vi "YENİİİİİ.vi"() -> ()   [LabVIEW 2018]
uses:
  <vilib>/Instr/_visa.llb/VISA Configure Serial Port (Instr).vi
panel:
  out "humimade":dbl(knob) scale=0.0..100.0
  out "temperature":dbl(slide) scale=0.0..100.0
  out "humimade":i32
  in  "stop":bool
  out "termo":i32
  in  "VISA resource name":refnum<visa-resource-name>
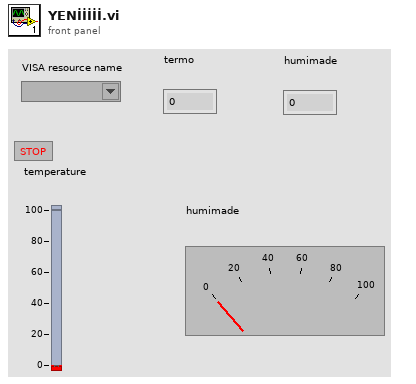
[diagram p1: front panel]
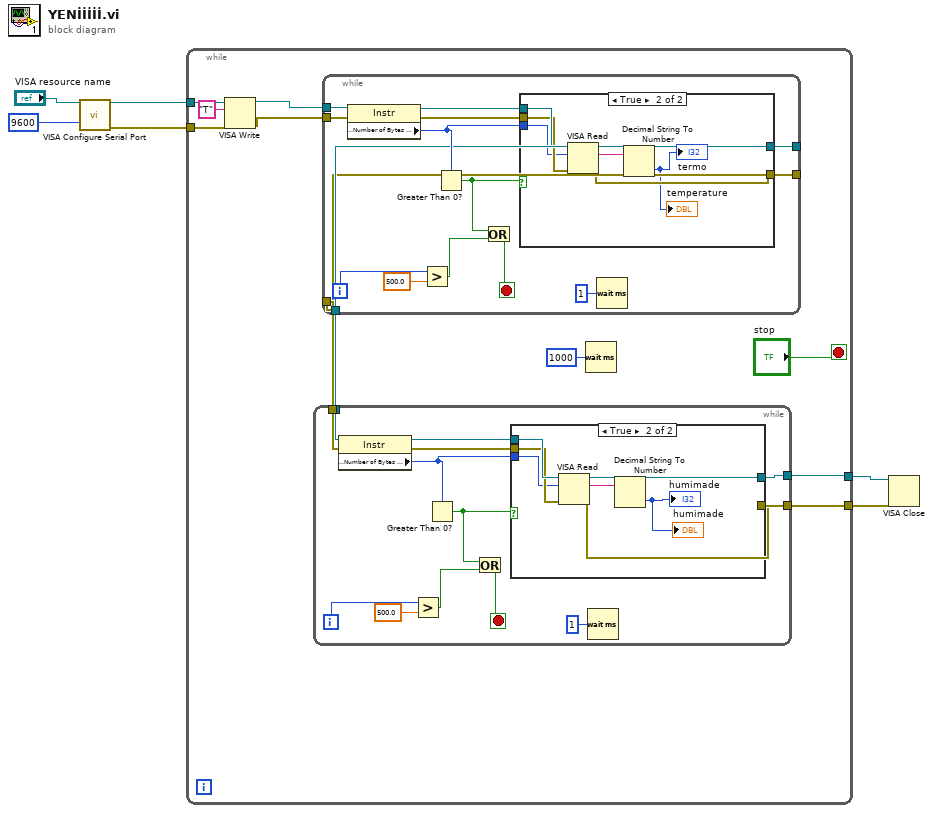
[diagram p0: block diagram]
diagram:
  n1 = call-poly "VISA Configure Serial Port"("VISA resource name"="VISA resource name", "baud rate (9600)"=u32 9600) -> ("VISA resource name out"=w4:refnum<visa-resource-name>, "error out"=w3:errorcluster)  [unwired: 12 in]
  n2 = while {
    tunnel: w4 -> [w17]
    tunnel: w3 -> [w16]
    tunnel: [w10] -> w2
    tunnel: [w9] -> w1
    stop <- "stop" stop-if-true
    n3 = VISA Write(VISA resource name=w17, write buffer="T", error in (no error)=w16) -> (VISA resource name out=w14:refnum<visa-resource-name>, error out=w13:errorcluster)  [unwired: 1 out]
    n4 = while {
      tunnel: w14 -> [w52]
      tunnel: w13 -> [w51]
      tunnel: [w41] -> _
      tunnel: [w40] -> _
      tunnel: [w41] -> w8
      tunnel: [w40] -> w7
      i -> [w45]
      stop <- w43 stop-if-true
      n5 = property class="Instr"(reference=w52, error in=w51) -> (reference out=w50:refnum<visa-resource-name>, error out=w49:errorcluster, "Serial Settings:Number of Bytes at Serial Port"=w48:u32)
      n6 = Greater?(x=w45, y=500.0) -> (0:w47:bool)
      n7 = Greater Than 0?(x=w48) -> (x > 0?=w44:bool)
      n8 = Or(x=w44, y=w47) -> (x .or. y?=w43:bool)
      n9 = case shown="True" w44 {
        tunnel: w50 -> [w54 w61]
        tunnel: w49 -> [w53 w60]
        tunnel: w48 -> [_ w59]
        tunnel: [w54 w57] -> w41
        tunnel: [w53 w56] -> w40
        frame False {
        }
        frame True {
          n10 = VISA Read(VISA resource name=w61, byte count=w59, error in (no error)=w60) -> (VISA resource name out=w57:refnum<visa-resource-name>, read buffer=w58:string, error out=w56:errorcluster)  [unwired: 1 out]
          n11 = Decimal String To Number(string=w58) -> (number=→"termo" →"temperature":i32)  [unwired: 2 in, 1 out]
        }
      }
      n12 = Wait (ms)(milliseconds to wait=u32 1) -> ()  [unwired: 1 out]
    }
    n13 = while {
      tunnel: [w27] -> w10
      tunnel: [w26] -> w9
      tunnel: w8 -> [w19]
      tunnel: w7 -> [w18]
      i -> [w23]
      stop <- w21 stop-if-true
      n14 = property class="Instr"(reference=w19, error in=w18) -> (reference out=w30:refnum<visa-resource-name>, error out=w29:errorcluster, "Serial Settings:Number of Bytes at Serial Port"=w28:u32)
      n15 = Greater?(x=w23, y=500.0) -> (0:w25:bool)
      n16 = Greater Than 0?(x=w28) -> (x > 0?=w22:bool)
      n17 = Or(x=w22, y=w25) -> (x .or. y?=w21:bool)
      n18 = case shown="True" w22 {
        tunnel: w30 -> [w32 w39]
        tunnel: w29 -> [w31 w38]
        tunnel: w28 -> [_ w37]
        tunnel: [w32 w35] -> w27
        tunnel: [w31 w34] -> w26
        frame False {
        }
        frame True {
          n19 = VISA Read(VISA resource name=w39, byte count=w37, error in (no error)=w38) -> (VISA resource name out=w35:refnum<visa-resource-name>, read buffer=w36:string, error out=w34:errorcluster)  [unwired: 1 out]
          n20 = Decimal String To Number(string=w36) -> (number=→"humimade" →"humimade":i32)  [unwired: 2 in, 1 out]
        }
      }
      n21 = Wait (ms)(milliseconds to wait=u32 1) -> ()  [unwired: 1 out]
    }
    n22 = Wait (ms)(milliseconds to wait=u32 1000) -> ()  [unwired: 1 out]
  }
  n23 = VISA Close(VISA resource name=w2, error in (no error)=w1) -> ()  [unwired: 1 out]
